vi "Open Database Connection.vi"(8 "error in (no error)":errorcluster, 10 "Initialize DatabaseQueue":bool, 11 "AcquistionObject in":refnum<class "AcquistionObject.lvclass">) -> (0 "error out":errorcluster, 3 "AcquistionObject out":refnum<class "AcquistionObject.lvclass">)   [LabVIEW 2012, in "AcquisitionCoreObjects.lvlib" / "AcquistionObject.lvclass"]
uses:
  AcquistionObject.lvclass
  <vilib>/addons/database/Connection.llb/Conn ObjectReference.ctl
  AcquistionObject.lvclass/AcquistionObject.ctl
  <vilib>/Utility/config.llb/Read Key (Path).vi
  <vilib>/Utility/config.llb/Read Key (String).vi
  <vilib>/addons/database/Connection.llb/DB Tools Open Connec (Path).vi
  <vilib>/Utility/config.llb/NI_LVConfig.lvlib
  <vilib>/addons/database/NI_Database_API.lvlib
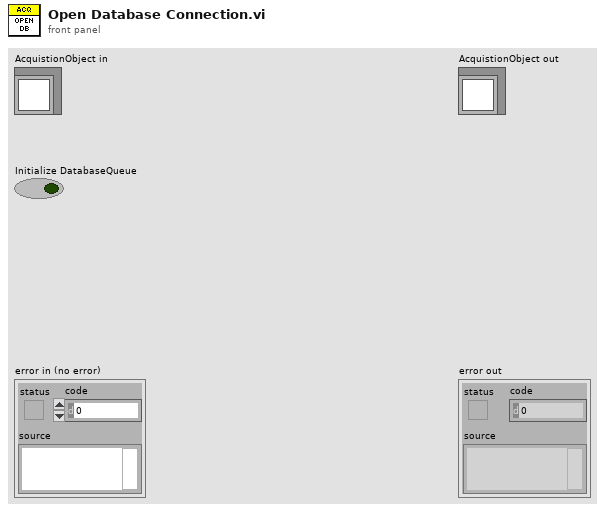
[diagram p1: front panel]
types:
  T1 = typedef "NI_Database_API.lvlib/Conn ObjectReference.ctl" = refnum<k1>
  T2 = cluster{cluster{"reference":T1, "table":string, "columns":string[], i32}, "Variant":variant}
  T3 = typedef "NI_LVConfig.lvlib/Config Data RefNum.ctl" = refnum<k1>
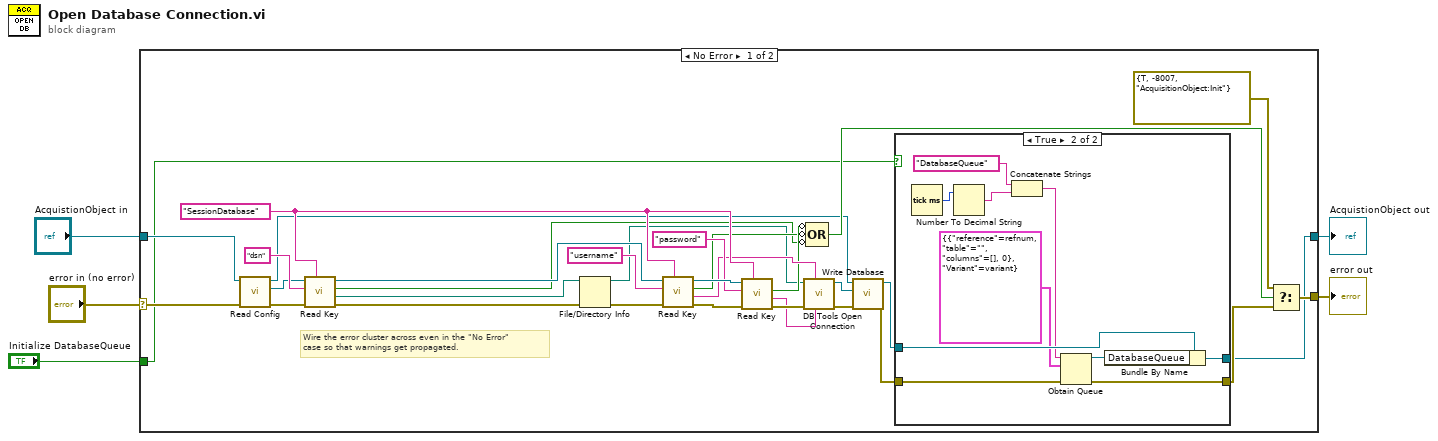
[diagram p0: block diagram]
diagram:
  n1 = case shown="No Error" "error in (no error)" {
    selector: "error in (no error)" -> [w13 w51]
    tunnel: [w12 w51] -> w2
    tunnel: [w6 w50] -> w5
    tunnel: "AcquistionObject in" -> [w18 w50]
    tunnel: "Initialize DatabaseQueue" -> [w8 _]
    frame No Error {
      w29 = "SessionDatabase" ("section")
      # "Wire the error cluster across even in the \"No Error\"\ncase so that warnings get propagated."
      n2 = call-dynamic "Read Config.vi"("error in (no error)"=w13, "AcquistionObject in"=w18) -> ("error out"=w19:errorcluster, "config data"=w36:T3, "AcquistionObject out"=w11:refnum<class "AcquistionObject.lvclass">)  [unwired: 7 in]
      n3 = call-poly <vilib>:"Read Key.vi"("section"=w29, "error in (no error)"=w19, "key"="dsn", "refnum"=w36) -> ("error out"=w23:errorcluster, "value"=w21:path, "found?"=w24:bool, "refnum out"=w35:T3)  [unwired: 4 in]
      n4 = File/Directory Info(path=w21, error in=w23) -> (path out=w20:path, error out=w22:errorcluster)  [unwired: 5 out]
      n5 = call-poly <vilib>:"Read Key.vi"("section"=w29, "error in (no error)"=w22, "key"="username", "refnum"=w35) -> ("error out"=w33:errorcluster, "value"=w28:string, "found?"=w25:bool, "refnum out"=w32:T3)  [unwired: 4 in]
      n6 = call-poly <vilib>:"Read Key.vi"("section"=w29, "error in (no error)"=w33, "key"="password", "refnum"=w32) -> ("error out"=w30:errorcluster, "value"=w27:string, "found?"=w26:bool)  [unwired: 4 in, 1 out]
      n7 = call-poly <vilib>:"DB Tools Open Connection.vi"("password"=w27, "userID"=w28, "error in (no error)"=w30, "connection information"=w20) -> ("error out"=w15:errorcluster, "connection reference"=w16:T1)  [unwired: 4 in]
      n8 = Compound Arithmetic op=OR(invert w26, invert w25, invert w24) -> (w14:bool)
      n9 = call-dynamic "Write Database.vi"("error in (no error)"=w15, "reference"=w16, "AcquistionObject in"=w11) -> ("error out"=w10:errorcluster, "AcquistionObject out"=w7:refnum<class "AcquistionObject.lvclass">)  [unwired: 7 in]
      n10 = case shown="True" w8 {
        tunnel: w10 -> [w39 w49]
        tunnel: [w39 w48] -> w9
        tunnel: w7 -> [w38 w46]
        tunnel: [w38 w45] -> w6
        frame False {
        }
        frame True {
          n11 = Tick Count (ms)() -> (millisecond timer value=w41:u32)
          n12 = Number To Decimal String(number=w41) -> (decimal integer string=w40:string)  [unwired: 1 in]
          n13 = Concatenate Strings("DatabaseQueue" ("name (unnamed)"), w40) -> (w42:string)
          n14 = Obtain Queue(name (unnamed)=w42, element data type=T2 {{"reference"=refnum, "table"="", "columns"=[], 0}, "Variant"=variant} ("output cluster"), error in (no error)=w49) -> (queue out=w47:refnum<queue>, error out=w48:errorcluster)  [unwired: 2 in, 1 out]
          n15 = Bundle By Name(cluster=w46, "DatabaseQueue"=w47) -> (w45:refnum<class "AcquistionObject.lvclass">)
        }
      }
      n16 = Select(t=errorcluster {"status"=TRUE, "code"=-8007, "source"="AcquisitionObject:Init"}, s=w14, f=w9) -> (s? t:f=w12:errorcluster)
    }
    frame Error {
    }
  }
  "error out" <- w2
  "AcquistionObject out" <- w5
